vi "sine_fitting.vi"(6 "Sampling Frequency [Hz]":dbl, 10 "Frequency [Hz]":dbl, 11 "RX data":dbl[](array[numeric])) -> (2 "DC Offset":dbl, 3 "Amplidude":dbl)   [LabVIEW 2025, in "LabJackEKG.lvlib"]
uses:
  LabJackEKG.lvlib
  <vilib>/Analysis/NI_AALPro.lvlib
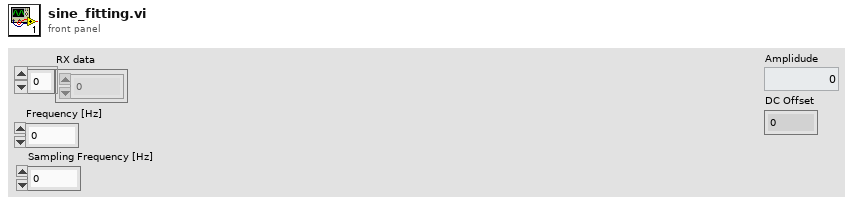
[diagram p1: front panel]
types:
  T1 = enum32{"do not compute Covariance", " compute Covariance"}
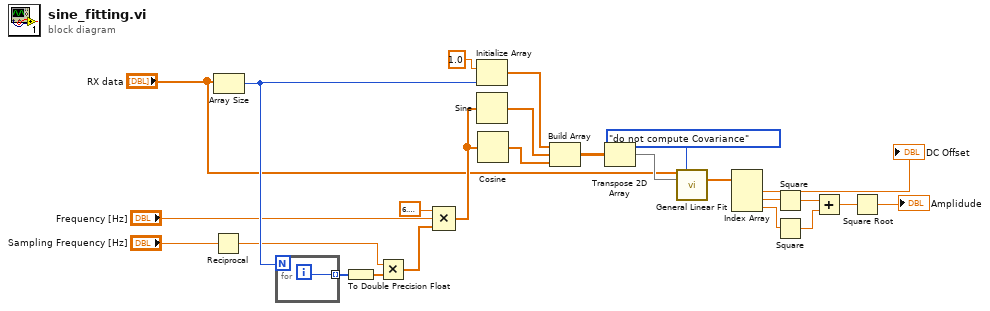
[diagram p0: block diagram]
diagram:
  n1 = Reciprocal(x="Sampling Frequency [Hz]") -> (1/x=w1:dbl)
  n2 = Array Size(array="RX data") -> (size(s)=w10:i32)
  n3 = for {
    N: w10 -> [_]
    tunnel: [w26] -> w9 mode=indexing
    i -> [w26]
  }
  n4 = To Double Precision Float(number=w9) -> (double precision float=w8:dbl[])
  n5 = Multiply(x=w1, y=w8) -> (x*y=w6:dbl[])
  n6 = Compound Arithmetic op=MULTIPLY(6.283185307179586, "Frequency [Hz]", w6) -> (w25:dbl[])
  n7 = Initialize Array(1.0 ("element"), w10) -> (w23:dbl[])
  n8 = Sine(x=w25) -> (sin(x)=w21:dbl[])
  n9 = Cosine(x=w25) -> (cos(x)=w20:dbl[])
  n10 = Build Array(w23, w21, w20) -> (w22:dbl[][])
  n11 = Transpose 2D Array(2D array=w22) -> (transposed array=w19:dbl[][])
  n12 = call <vilib>:"General Linear Fit.vi"("Y"="RX data", "covariance selector"=T1."do not compute Covariance", "H"=w19) -> ("Coefficients"=w12:dbl[])  [unwired: 7 in, 5 out]
  n13 = Index Array(array=w12) -> (element #1=→"DC Offset":dbl, element #2=w17:dbl, element #3=w16:dbl)  [unwired: 3 in]
  n14 = Square(x=w17) -> (x^2=w15:dbl)
  n15 = Square(x=w16) -> (x^2=w14:dbl)
  n16 = Add(x=w15, y=w14) -> (x+y=w13:dbl)
  n17 = Square Root(x=w13) -> (sqrt(x)=→"Amplidude":dbl)
